vi "init.vi"() -> ()   [LabVIEW 2018]
panel:
  in  "String 3":string caption="String"
  in  "String 2":string caption="String"
  in  "String":string
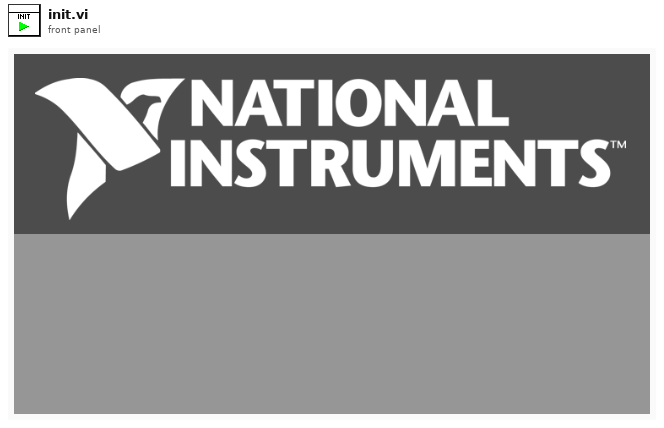
[diagram p1: front panel]
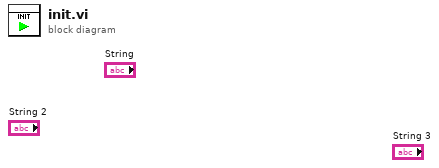
[diagram p0: block diagram]
diagram:
